vi "Symmetrize (single).vi"(8 "error in (no error)":errorcluster, 11 "XY-data":cluster{"X-array":dbl[], "Y-array":dbl[]} {"Y-array" format="%.2p"; "X-array" format="%.2p"}) -> (0 "error out":errorcluster, 1 "Antisymmetric":cluster{"X-array":dbl[], dbl[]}, 2 "Symmetric":cluster{"X-array":dbl[], dbl[]}, 3 "XY-data out":cluster{"X-array":dbl[], "Y-array":dbl[]} {"Y-array" format="%.2p"; "X-array" format="%.2p"})   [LabVIEW 2019, in "xy_utilities.lvlib"]
doc: "Compute the Symmetric and Antisymmetric functions of <b>XY-data</b>\n\n<b>Symmetric</b>: f+ = (f(x) + f(-x))/2\n<b>Antisymmetric</b>: f- = (f(x) - f(-x))/2"
uses:
  xy_utilities.lvlib
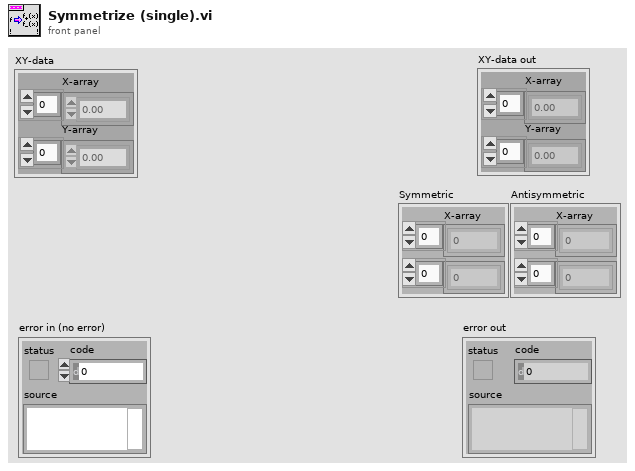
[diagram p1: front panel]
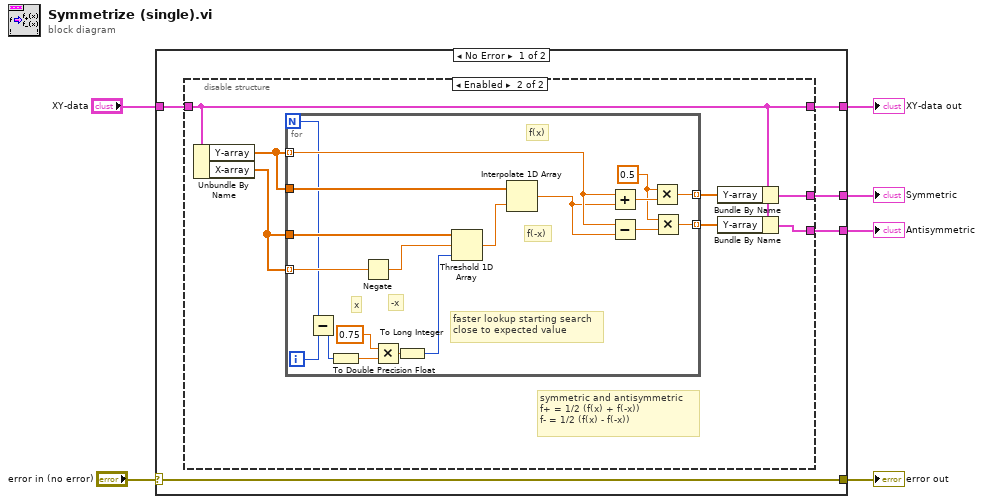
[diagram p0: block diagram]
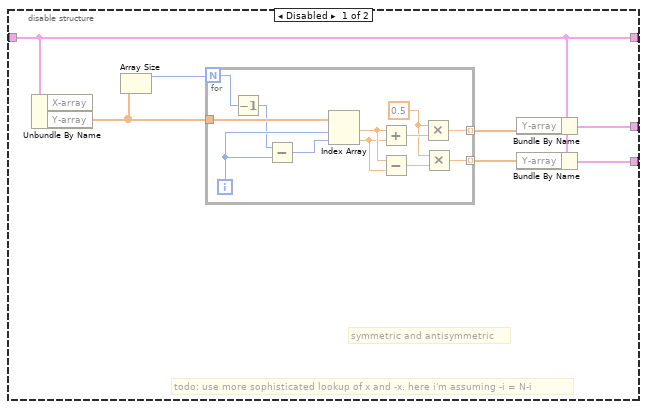
[diagram p2: hidden frame]
diagram:
  n1 = case shown="No Error" "error in (no error)" {
    selector: "error in (no error)" -> [w11 w58]
    tunnel: [w11 w58] -> w5
    tunnel: "XY-data" -> [w10 w57]
    tunnel: [w7 w57] -> w3
    tunnel: [w9 _] -> w2
    tunnel: [w8 _] -> w1
    frame No Error {
      n2 = disable-structure shown="Enabled" {
        disable-tunnel: w10 -> [w14 w34]
        disable-tunnel: [w13 w36] -> w9
        disable-tunnel: [w12 w35] -> w8
        disable-tunnel: [w14 w34] -> w7
        frame Disabled {
          # "symmetric and antisymmetric"
          # "todo: use more sophisticated lookup of x and -x. here i'm assuming -i = N-i"
          n3 = Unbundle By Name(w14) -> ("Y-array"=w15:dbl[])  [unwired: 1 out]
          n4 = Array Size(array=w15) -> (size(s)=w16:i32)
          n5 = for {
            N: w16 -> [w20]
            tunnel: w15 -> [w30]
            tunnel: [w23] -> w17 mode=indexing
            tunnel: [w22] -> w18 mode=indexing
            i -> [w29]
            w24 = 0.5 ("x")
            n6 = Decrement(x=w20) -> (x-1=w21:i32)
            n7 = Subtract(x=w21, y=w29) -> (x-y=w19:i32)
            n8 = Index Array(array=w30, index #1=w29, index #2=w19) -> (element #1=w28:dbl, element #2=w27:dbl)
            n9 = Add(x=w28, y=w27) -> (x+y=w26:dbl)
            n10 = Subtract(x=w28, y=w27) -> (x-y=w25:dbl)
            n11 = Multiply(x=w24, y=w26) -> (x*y=w23:dbl)
            n12 = Multiply(x=w24, y=w25) -> (x*y=w22:dbl)
          }
          n13 = Bundle By Name(cluster=w14, "Y-array"=w17) -> (w13:cluster{"X-array":dbl[], "Y-array":dbl[]})
          n14 = Bundle By Name(cluster=w14, "Y-array"=w18) -> (w12:cluster{"X-array":dbl[], "Y-array":dbl[]})
        }
        frame Enabled {
          # "symmetric and antisymmetric\nf+ = 1/2 (f(x) + f(-x))\nf- = 1/2 (f(x) - f(-x))"
          n15 = Unbundle By Name(w34) -> ("Y-array"=w32:dbl[], "X-array"=w33:dbl[])
          n16 = for {
            N -> [w44]
            tunnel: [w47] -> w37 mode=indexing
            tunnel: [w46] -> w31 mode=indexing
            tunnel: w33 -> [w56] mode=indexing
            tunnel: w33 -> [w55]
            tunnel: w32 -> [w52]
            tunnel: w32 -> [w48] mode=indexing
            i -> [w43]
            w49 = 0.5 ("x")
            # "faster lookup starting search\nclose to expected value"
            # "f(x)"
            # "x"
            # "f(-x)"
            # "-x"
            n17 = Subtract(x=w44, y=w43) -> (x-y=w41:i32)
            n18 = To Double Precision Float(number=w41) -> (double precision float=w38:dbl)
            n19 = Negate(x=w56) -> (-x=w54:dbl)
            n20 = Multiply(x=0.75, y=w38) -> (x*y=w40:dbl)
            n21 = To Long Integer(number=w40) -> (32bit integer=w39:i32)
            n22 = Threshold 1D Array(1:w39, 2:w54, 3:w55) -> (0:w53:dbl)
            n23 = Interpolate 1D Array(1:w53, 2:w52) -> (0:w45:dbl)
            n24 = Add(x=w48, y=w45) -> (x+y=w51:dbl)
            n25 = Subtract(x=w48, y=w45) -> (x-y=w50:dbl)
            n26 = Multiply(x=w49, y=w51) -> (x*y=w47:dbl)
            n27 = Multiply(x=w49, y=w50) -> (x*y=w46:dbl)
          }
          n28 = Bundle By Name(cluster=w34, "Y-array"=w37) -> (w36:cluster{"X-array":dbl[], "Y-array":dbl[]})
          n29 = Bundle By Name(cluster=w34, "Y-array"=w31) -> (w35:cluster{"X-array":dbl[], "Y-array":dbl[]})
        }
      }
    }
    frame Error {
    }
  }
  "error out" <- w5
  "XY-data out" <- w3
  "Symmetric" <- w2
  "Antisymmetric" <- w1
